vi "Replace -.vi"(10 "Numeric":i32, 11 "Array in":string[][](array[string])) -> (3 "Array out":string[][](array[string]))   [LabVIEW 2021]
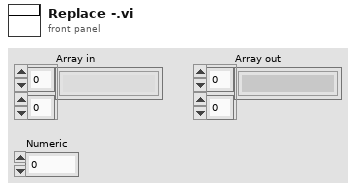
[diagram p1: front panel]
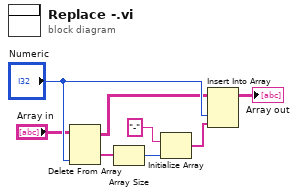
[diagram p0: block diagram]
diagram:
  n1 = Delete From Array(array="Array in", index (col)="Numeric") -> (deleted portion=w2:string[], array with subset deleted=w5:string[][])  [unwired: 2 in]
  n2 = Array Size(array=w2) -> (size(s)=w3:i32)
  n3 = Initialize Array("-", w3) -> (w4:string[])
  n4 = Insert Into Array(array=w5, index (col)="Numeric", new element=w4) -> (→"Array out":string[][])  [unwired: 1 in]
